vi "create scan vectr.vi"(1 "Table Control":string[][](table), 2 "waypoint mode?":bool=TRUE) -> (0 "Array":dbl[](array[numeric]))   [LabVIEW 2015]
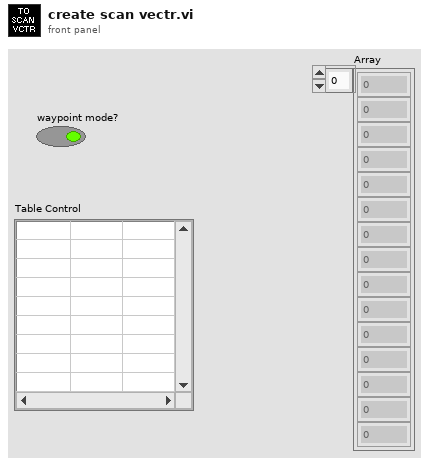
[diagram p1: front panel]
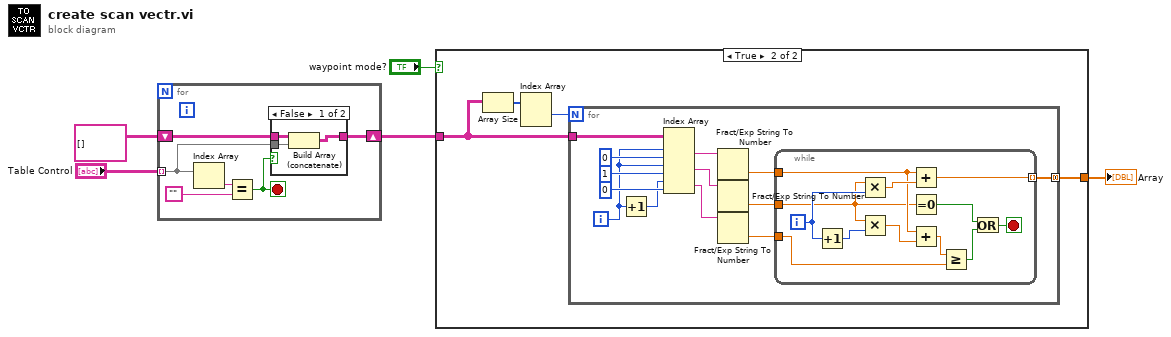
[diagram p0: block diagram]
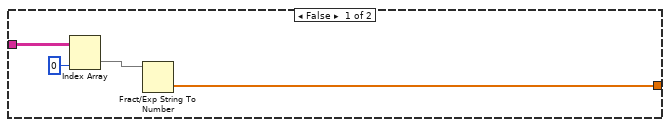
[diagram p2: hidden frame]
diagram:
  n1 = for {
    tunnel: "Table Control" -> [w7] mode=indexing
    shift-right: [w6] -> w2
    shift-left: string[][] [] ("t") -> [w9]
    stop <- w8 stop-if-true
    n2 = Index Array(array=w7) -> (element=w10:string)  [unwired: 1 in]
    n3 = Equal?(x=w10, y="") -> (x = y?=w8:bool)
    n4 = case shown="False" w8 {
      tunnel: w9 -> [w14 w15]
      tunnel: w7 -> [w13 _]
      tunnel: [w12 w15] -> w6
      frame False {
        n5 = Build Array (concatenate)(w14, w13) -> (w12:string[][])
      }
      frame True {
      }
    }
  }
  n6 = case shown="True" "waypoint mode?" {
    tunnel: [w17 w21] -> w3
    tunnel: w2 -> [w18 w20]
    frame False {
      n7 = Index Array(array=w18, index (col)=0 ("disabled index (col)")) -> (element=w19:string[])  [unwired: 1 in]
      n8 = Fract/Exp String To Number(string=w19) -> (number=w17:dbl[])  [unwired: 3 in, 1 out]
    }
    frame True {
      n9 = Array Size(array=w20) -> (size(s)=w23:i32[])
      n10 = Index Array(array=w23) -> (element #1=w22:i32)  [unwired: 2 in, 1 out]
      n11 = for {
        N: w22 -> [_]
        tunnel: w20 -> [w32]
        tunnel: [w24] -> w21 mode=concatenating
        i -> [w31]
        n12 = Increment(x=w31) -> (x+1=w34:i32)
        n13 = Index Array(array=w32, index (row) #1=w31, index (col) #1=0 ("disabled index (col)"), index (row) #2=w31, index (col) #2=1 ("disabled index (col)"), index (row) #3=w34, index (col) #3=0 ("disabled index (col)")) -> (element #1=w30:string, element #2=w29:string, element #3=w28:string)
        n14 = Fract/Exp String To Number(string=w30) -> (number=w27:dbl)  [unwired: 3 in, 1 out]
        n15 = Fract/Exp String To Number(string=w29) -> (number=w26:dbl)  [unwired: 3 in, 1 out]
        n16 = Fract/Exp String To Number(string=w28) -> (number=w25:dbl)  [unwired: 3 in, 1 out]
        n17 = while {
          tunnel: w27 -> [w43]
          tunnel: w26 -> [w40]
          tunnel: w25 -> [w41]
          tunnel: [w47] -> w24 mode=indexing
          i -> [w45]
          stop <- w37 stop-if-true
          n18 = Increment(x=w45) -> (x+1=w44:i32)
          n19 = Multiply(x=w40, y=w45) -> (x*y=w48:dbl)
          n20 = Multiply(x=w40, y=w44) -> (x*y=w46:dbl)
          n21 = Add(x=w43, y=w48) -> (x+y=w47:dbl)
          n22 = Equal To 0?(x=w40) -> (x = 0?=w39:bool)
          n23 = Add(x=w43, y=w46) -> (x+y=w42:dbl)
          n24 = Greater Or Equal?(x=w42, y=w41) -> (x >= y?=w38:bool)
          n25 = Or(x=w39, y=w38) -> (x .or. y?=w37:bool)
        }
      }
    }
  }
  "Array" <- w3
